vi "Change Pin.vi"(6 "Cache in":u16 format="%.0b", 7 "Pin":T4 min=1 max=16, 8 "error in (no error)":errorcluster, 9 "Value":u8 format="%.0b", 10 "Reg Address":T2, 11 "Chip Address (A2 A1 A0)":T3 max=7) -> (0 "error out":errorcluster, 3 "SPI Command":T1, 4 "Cache out":u16 format="%.0b")   [LabVIEW 2014, in "SLSC configuration Shared.lvlib"]
doc: "Changes an individual pin on the desired register address in sequential mode. This VI requires the previous value of the register and subsequent register."
uses:
  SLSC configuration Shared.lvlib
  Pin.ctl
  Chip Address.ctl
  IOCON BANK 0 Reg Addresses.ctl
  SPI Command.ctl
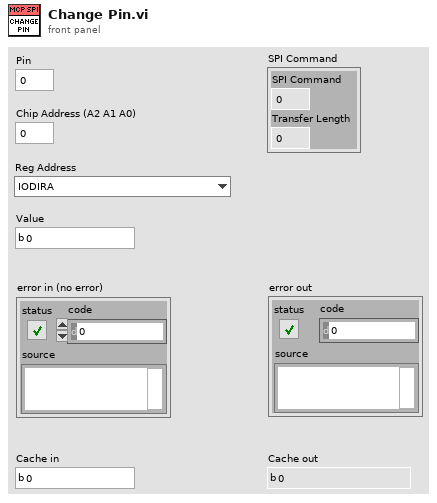
[diagram p1: front panel]
types:
  T1 = typedef "SLSC configuration Shared.lvlib/SPI Command.ctl" = cluster{"SPI Command":u32, "Transfer Length":u8}
  T2 = typedef "SLSC configuration Shared.lvlib/IOCON BANK 0 Reg Addresses.ctl" = enum8{"IODIRA", "IODIRB", "IPOLA", "IPOLB", "GPINTENA", "GPINTENB", "DEFVALA", "DEFVALB", "INTCONA", "INTCONB", "IOCONA", "IOCONB", "GPPUA", "GPPUB", "INTFA", "INTFB", "INTCAPA", "INTCAPB", "GPIOA", "GPIOB", "OLATA", "OLATB"}
  T3 = typedef "SLSC configuration Shared.lvlib/Chip Address.ctl" = u8
  T4 = typedef "SLSC configuration Shared.lvlib/Pin.ctl" = u8
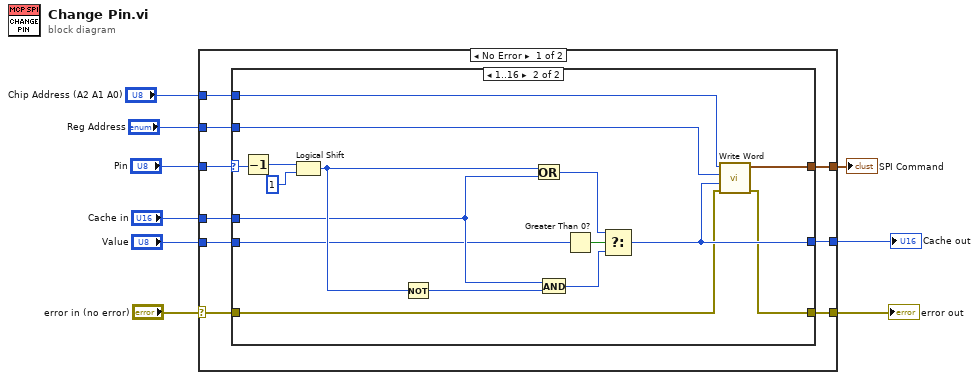
[diagram p0: block diagram]
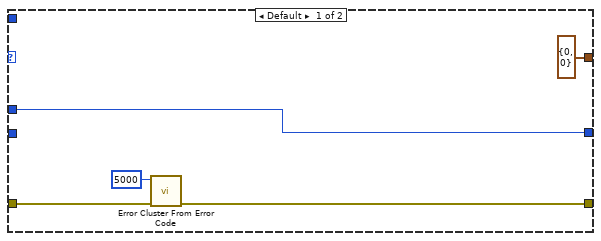
[diagram p2: hidden frame]
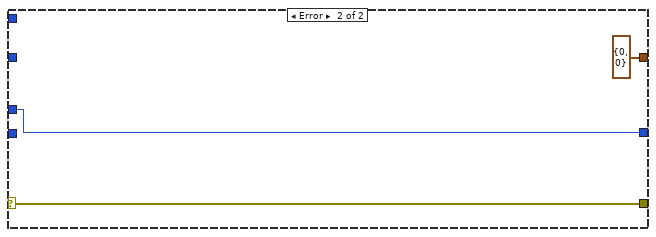
[diagram p3: hidden frame]
diagram:
  n1 = case shown="No Error" "error in (no error)" {
    selector: "error in (no error)" -> [w10 w42]
    tunnel: [w18 w41] -> w9
    tunnel: [w17 T1 {"SPI Command"=0, "Transfer Length"=0} ("SPI Command")] -> w1
    tunnel: "Pin" -> [w16 _]
    tunnel: "Cache in" -> [w15 w41]
    tunnel: "Value" -> [w14 _]
    tunnel: [w13 w42] -> w5
    tunnel: "Reg Address" -> [w12 _]
    tunnel: "Chip Address (A2 A1 A0)" -> [w11 _]
    frame No Error {
      n2 = case shown="1..16" w16 {
        selector: w16 -> [_ w30]
        tunnel: [w23 w39] -> w18
        tunnel: [T1 {"SPI Command"=0, "Transfer Length"=0} ("SPI Command") w31] -> w17
        tunnel: w15 -> [w23 w29]
        tunnel: w14 -> [_ w28]
        tunnel: [w21 w24] -> w13
        tunnel: w12 -> [_ w27]
        tunnel: w11 -> [_ w26]
        tunnel: w10 -> [w20 w25]
        frame Default {
          n3 = call <vilib>:"Error Cluster From Error Code.vi"("error in (no error)"=w20, "error code (0)"=5000) -> ("error out"=w21:errorcluster)  [unwired: 7 in]
        }
        frame 1..16 {
          n4 = Decrement(x=w30) -> (x-1=w32:T4)
          n5 = Logical Shift(y=w32, x=u16 1) -> (x << y=w36:u16)
          n6 = Not(x=w36) -> (.not. x?=w37:u16)
          n7 = Or(x=w36, y=w29) -> (x .or. y?=w35:u16)
          n8 = And(x=w29, y=w37) -> (x .and. y?=w38:u16)
          n9 = Greater Than 0?(x=w28) -> (x > 0?=w34:bool)
          n10 = Select(t=w35, s=w34, f=w38) -> (s? t:f=w39:u16)
          n11 = call "Write Word.vi"("error in (no error)"=w25, "Value"=w39, "Reg Address"=w27, "Chip Address (A2 A1 A0)"=w26) -> ("error out"=w24:errorcluster, "SPI Command"=w31:T1)  [unwired: 6 in]
        }
      }
    }
    frame Error {
    }
  }
  "Cache out" <- w9
  "error out" <- w5
  "SPI Command" <- w1
